vi "uninstall.vi"(8 "error in (no error)":errorcluster, 11 "plugin_interface in":refnum<class "odbc_driver_postgres_v13.0.2.lvclass">) -> (0 "error out":errorcluster, 3 "plugin_interface out":refnum<class "odbc_driver_postgres_v13.0.2.lvclass">)   [LabVIEW 2015, in "lv-example-postgres-post-installer.lvlib" / "odbc_driver_postgres_v13.0.2.lvclass"]
uses:
  odbc_driver_postgres_v13.0.2.lvclass
  <userlib>/antonio-alexander/lv-bin-windows/public/api/v1/v1.lvlib
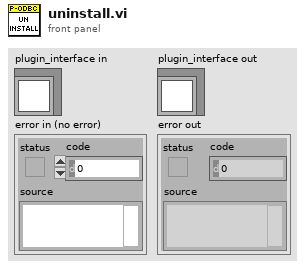
[diagram p1: front panel]
types:
  T1 = cluster{"display_name []":string[], "uninstall_string []":string[], "install_source []":string[], "install_location []":string[]}
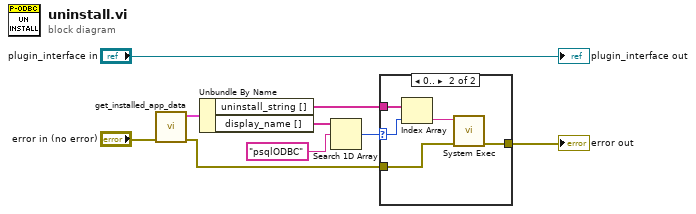
[diagram p0: block diagram]
diagram:
  n1 = call <userlib>:"get_installed_app_data.vi"("error in (no error)"="error in (no error)") -> ("error out"=w3:errorcluster, "installed_application_data []"=w4:T1)  [unwired: 9 in]
  n2 = Unbundle By Name(w4) -> ("uninstall_string []"=w6:string[], "display_name []"=w7:string[])
  n3 = Search 1D Array(1D array=w7, element="psqlODBC") -> (index of element=w5:i32)  [unwired: 1 in]
  n4 = case shown="0.." w5 {
    selector: w5 -> [_ w14]
    tunnel: w6 -> [_ w15]
    tunnel: w3 -> [w10 w12]
    tunnel: [w10 w11] -> w2
    frame Default {
    }
    frame 0.. {
      n5 = Index Array(array=w15, index=w14) -> (element=w13:string)
      n6 = call <vilib>:"System Exec.vi"("error in (no error)"=w12, "command line"=w13) -> ("error out"=w11:errorcluster)  [unwired: 6 in, 3 out]
    }
  }
  "error out" <- w2
  "plugin_interface out" <- "plugin_interface in"
